vi "RS232 485发送接收.vi"() -> ()   [LabVIEW 2010]
uses:
  全局量/全局_配置.vi
  <vilib>/Instr/_visa.llb/VISA Configure Serial Port (Instr).vi
panel:
  in  "单选_RS485_1":bool
  in  "单选_RS232_2":bool
  in  "单选_RS232_1":bool
  out "接收数据_3":string
  out "成功_3？":bool caption="成功？"
  in  "发送数据_3":string
  out "接收数据_2":string
  out "成功_2？":bool caption="成功？"
  in  "发送数据_2":string
  in  "btn_关闭":bool
  in  "btn_开始测试":bool
  out "接收数据_1":string
  out "成功_1？":bool caption="成功？"
  in  "发送数据_1":string
  # "RS232测试界面"
  # "1#发送字符"
  # "2#发送字符"
  # "1#接收字符"
  # "2#接收字符"
  # "1#测试结果"
  # "2#测试结果"
  # "RS485测试界面"
  # "1#发送字符"
  # "1#接收字符"
  # "1#测试结果"
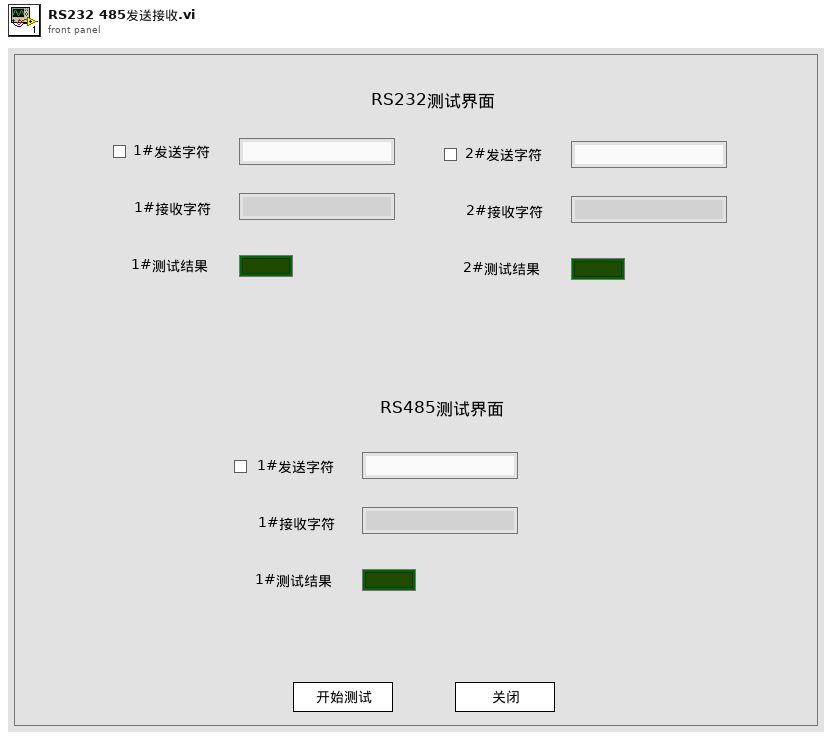
[diagram p1: front panel]
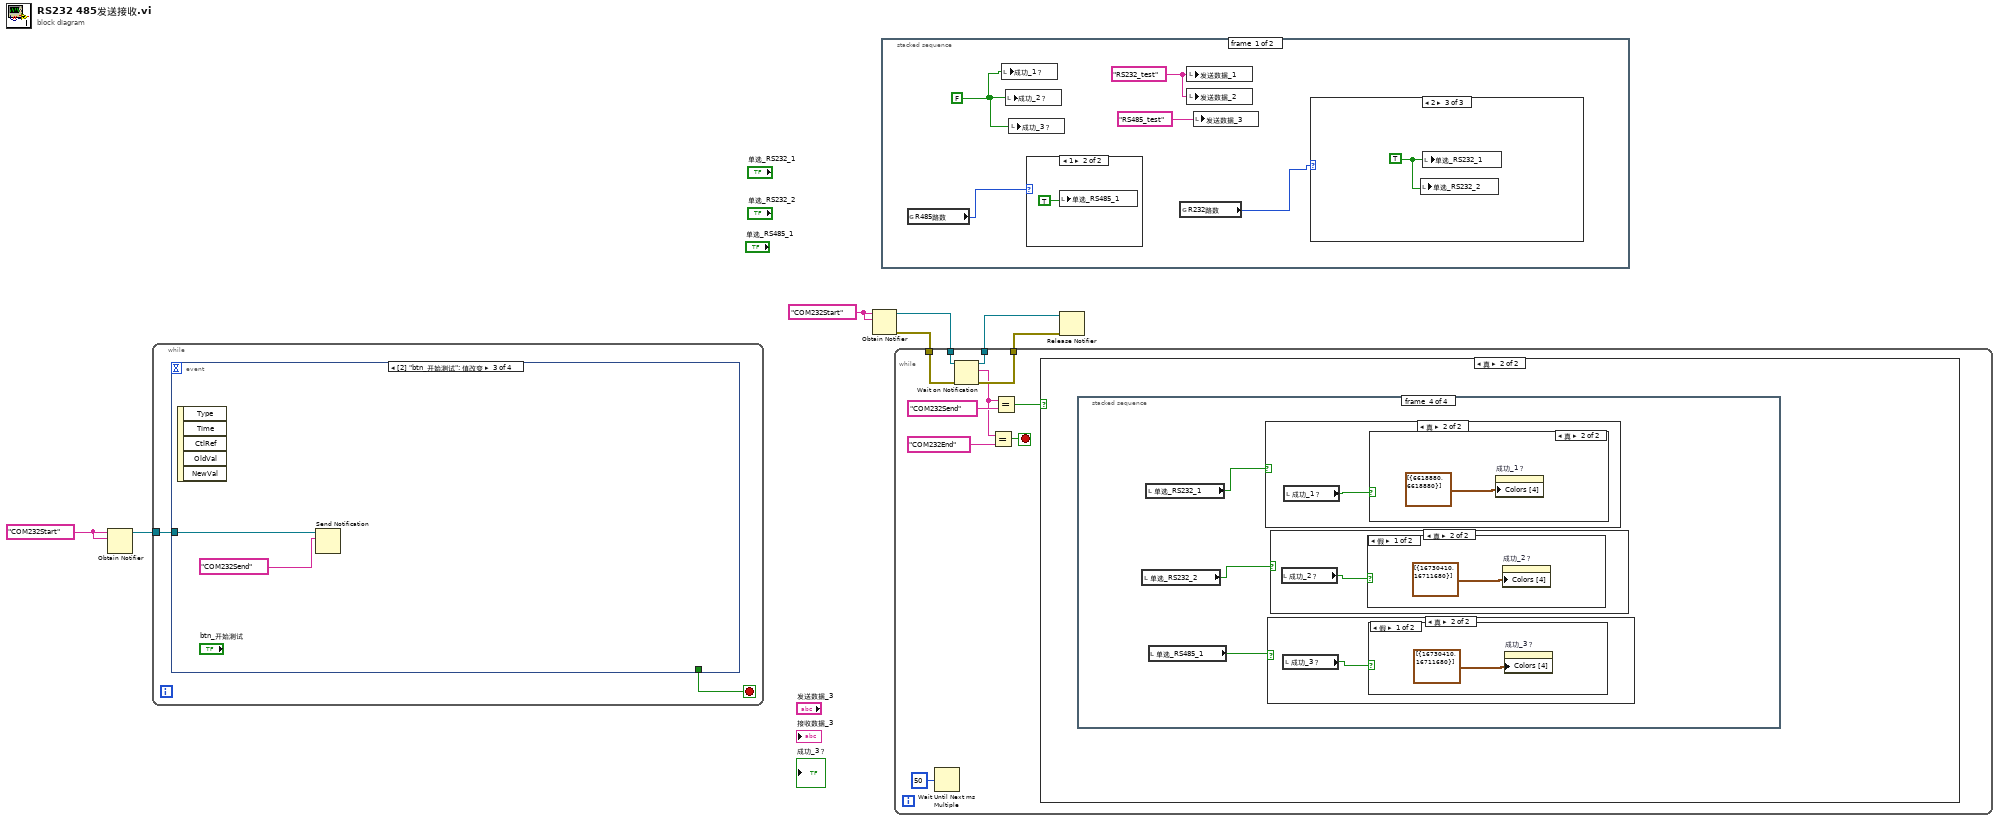
[diagram p0: block diagram]
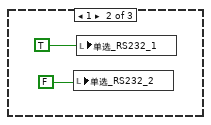
[diagram p3: hidden frame]
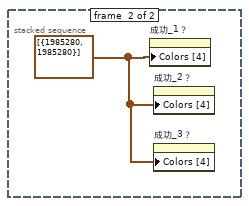
[diagram p5: hidden frame]
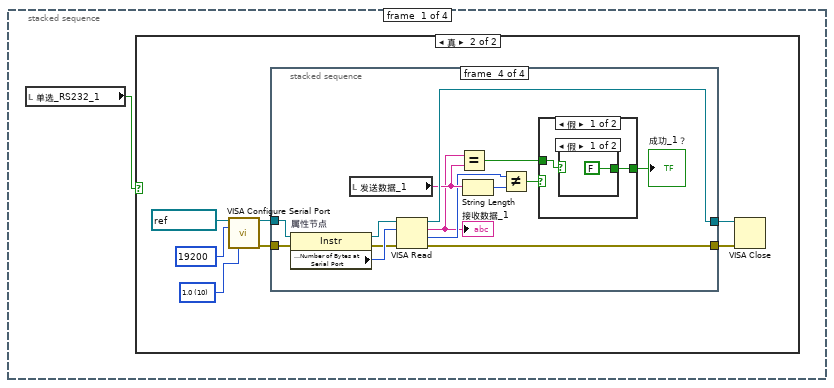
[diagram p7: hidden frame]
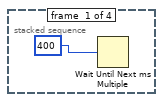
[diagram p9: hidden frame]
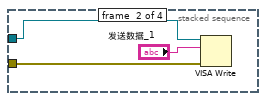
[diagram p10: hidden frame]
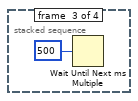
[diagram p11: hidden frame]
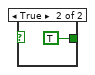
[diagram p12: hidden frame]
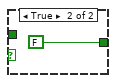
[diagram p13: hidden frame]
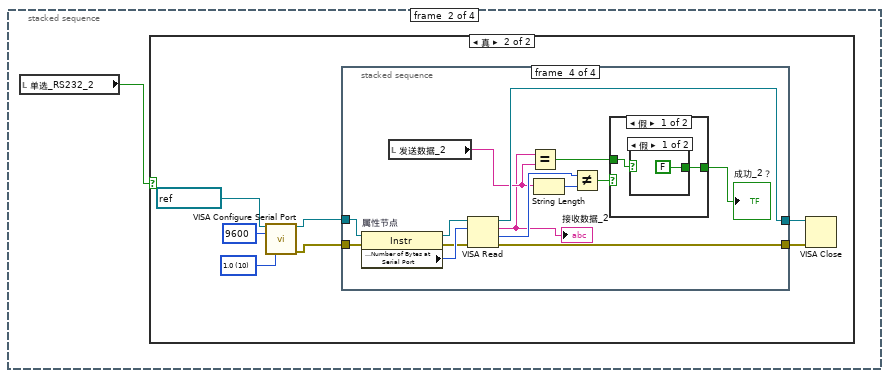
[diagram p14: hidden frame]
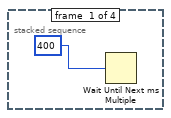
[diagram p16: hidden frame]
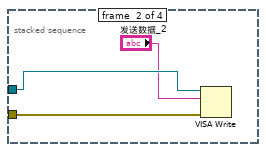
[diagram p17: hidden frame]
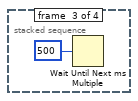
[diagram p18: hidden frame]
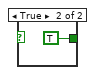
[diagram p19: hidden frame]
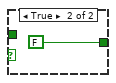
[diagram p20: hidden frame]
diagram:
  w2 = "COM232Start" ("名称（未命名）")
  w7 = "COM232Start" ("名称（未命名）")
  n1 = Obtain Notifier(name (unnamed)=w2, notification data type=w2) -> (notifier out=w1:refnum<notifier>)  [unwired: 2 in, 2 out]
  n2 = while {
    tunnel: w1 -> [w8]
    stop <- w9 stop-if-true
    n3 = event shown="[2] \"btn_开始测试\": 值改变" {
      selector: _ -> [_ _ _ _]
      dyn-events: _ -> [_ _ _ _]
      timeout: _ -> [_ _ _ _]
      tunnel: [_ TRUE _ TRUE] -> w9
      tunnel: w8 -> [_ w11 w13 w15]
      event Timeout {
        n4 = event-data() -> ()  [unwired: 1 in, 2 out]
      }
      event Panel Close {
        n5 = event-data() -> ()  [unwired: 1 in, 3 out]
        n6 = Send Notification(notification="COM232End" ("通知"), notifier=w11) -> ()  [unwired: 1 in, 2 out]
      }
      event "btn_开始测试": Value Change {
        n7 = event-data() -> ()  [unwired: 1 in, 5 out]
        n8 = Send Notification(notification="COM232Send" ("通知"), notifier=w13) -> ()  [unwired: 1 in, 2 out]
      }
      event "btn_关闭": Value Change {
        n9 = event-data() -> ()  [unwired: 1 in, 5 out]
        n10 = Send Notification(notification="COM232End" ("通知"), notifier=w15) -> ()  [unwired: 1 in, 2 out]
      }
    }
  }
  n11 = Obtain Notifier(name (unnamed)=w7, notification data type=w7) -> (notifier out=w6:refnum<notifier>, error out=w5:errorcluster)  [unwired: 2 in, 1 out]
  n12 = stacked-sequence {
    frame #0 {
      w20 = FALSE
      w22 = "RS232_test" ("发送数据_1")
      n13 = global read "全局_配置.vi" "R485路数"() -> (w18:u32)
      n14 = local write "成功_1？"(w20) -> ()
      n15 = local write "成功_2？"(w20) -> ()
      n16 = local write "成功_3？"(w20) -> ()
      n17 = case shown="1" w18 {
        frame 0, Default {
        }
        frame 1 {
          n18 = local write "单选_RS485_1"(TRUE) -> ()
        }
      }
      n19 = global read "全局_配置.vi" "R232路数"() -> (w19:u32)
      n20 = local write "发送数据_1"(w22) -> ()
      n21 = local write "发送数据_2"(w22) -> ()
      n22 = local write "发送数据_3"("RS485_test" ("发送数据_1")) -> ()
      n23 = case shown="2" w19 {
        frame 0, Default {
        }
        frame 1 {
          n24 = local write "单选_RS232_2"(FALSE) -> ()
          n25 = local write "单选_RS232_1"(TRUE) -> ()
        }
        frame 2 {
          w25 = TRUE
          n26 = local write "单选_RS232_2"(w25) -> ()
          n27 = local write "单选_RS232_1"(w25) -> ()
        }
      }
    }
    frame #1 {
      w27 = cluster{u32, u32}[] [{1985280, 1985280}]
      n28 = property on="成功_1？" class="Bool (严格)"("Colors [4]"=w27) -> ()  [unwired: 2 in, 2 out]
      n29 = property on="成功_2？" class="Bool (严格)"("Colors [4]"=w27) -> ()  [unwired: 2 in, 2 out]
      n30 = property on="成功_3？" class="Bool (严格)"("Colors [4]"=w27) -> ()  [unwired: 2 in, 2 out]
    }
  }
  n31 = while {
    tunnel: w6 -> [w37]
    tunnel: w5 -> [w36]
    tunnel: [w35] -> w4
    tunnel: [w34] -> w3
    stop <- w29 stop-if-true
    n32 = Wait Until Next ms Multiple(millisecond multiple=u32 50 ("毫秒倍数")) -> ()  [unwired: 1 out]
    n33 = Wait on Notification(notifier=w37, error in (no error)=w36) -> (notifier out=w35:refnum<notifier>, notification=w31:string, error out=w34:errorcluster)  [unwired: 2 in, 1 out]
    n34 = Equal?(x=w31, y="COM232End" ("通知")) -> (x = y?=w29:bool)
    n35 = Equal?(x=w31, y="COM232Send" ("通知")) -> (x = y?=w32:bool)
    n36 = case shown="真" w32 {
      frame False {
      }
      frame True {
        n37 = stacked-sequence {
          frame #0 {
            n38 = local read "单选_RS232_1"() -> (w38:bool)
            n39 = case shown="真" w38 {
              frame False {
              }
              frame True {
                w43 = u16 10 items=["1.0"=10, "1.5"=15, "2.0"=20] ("stop bits (10: 1 bit)")
                n40 = call-poly "VISA Configure Serial Port"("VISA resource name"=refnum<visa-resource-name> "COM1" ("R232端口"), "baud rate (9600)"=u32 19200, "stop bits (10: 1 bit)"=w43) -> ("VISA resource name out"=w42:refnum<visa-resource-name>, "error out"=w41:errorcluster)  [unwired: 11 in]
                n41 = stacked-sequence {
                  tunnel: w42 -> [_ w49 _ w62]
                  tunnel: w41 -> [_ w48 _ w61]
                  tunnel: [_ _ _ w64] -> w40
                  tunnel: [_ _ _ w63] -> w39
                  frame #0 {
                    n42 = Wait Until Next ms Multiple(millisecond multiple=u32 400 ("毫秒倍数")) -> ()  [unwired: 1 out]
                  }
                  frame #1 {
                    n43 = VISA Write(VISA resource name=w49, write buffer="发送数据_1", error in (no error)=w48) -> ()  [unwired: 3 out]
                  }
                  frame #2 {
                    n44 = Wait Until Next ms Multiple(millisecond multiple=u32 500 ("毫秒倍数")) -> ()  [unwired: 1 out]
                  }
                  frame #3 {
                    n45 = property on="属性节点" class="Instr"(reference=w62, error in=w61) -> (reference out=w58:refnum<visa-resource-name>, error out=w56:errorcluster, "Serial Settings:Number of Bytes at Serial Port"=w57:u32)
                    n46 = local read "发送数据_1"() -> (w55:string)
                    n47 = VISA Read(VISA resource name=w58, byte count=w57, error in (no error)=w56) -> (VISA resource name out=w64:refnum<visa-resource-name>, read buffer=w51:string, return count=w54:u32, error out=w63:errorcluster)
                    "接收数据_1" <- w51
                    n48 = Equal?(x=w51, y=w55) -> (x = y?=w60:bool)
                    n49 = String Length(string=w55) -> (length=w53:i32)
                    n50 = Not Equal?(x=w54, y=w53) -> (x != y?=w52:bool)
                    n51 = case shown="假" w52 {
                      tunnel: w60 -> [w66 _]
                      tunnel: [w65 FALSE] -> w59
                      frame False {
                        n52 = case shown="假" w66 {
                          tunnel: [FALSE TRUE] -> w65
                          frame False {
                          }
                          frame True {
                          }
                        }
                      }
                      frame True {
                      }
                    }
                    "成功_1？" <- w59
                  }
                }
                n53 = VISA Close(VISA resource name=w40, error in (no error)=w39) -> ()  [unwired: 1 out]
              }
            }
          }
          frame #1 {
            n54 = local read "单选_RS232_2"() -> (w70:bool)
            n55 = case shown="真" w70 {
              frame False {
              }
              frame True {
                w75 = u16 10 items=["1.0"=10, "1.5"=15, "2.0"=20] ("stop bits (10: 1 bit)")
                n56 = call-poly "VISA Configure Serial Port"("VISA resource name"=refnum<visa-resource-name> "COM3" ("R232端口"), "baud rate (9600)"=u32 9600, "stop bits (10: 1 bit)"=w75) -> ("VISA resource name out"=w72:refnum<visa-resource-name>, "error out"=w71:errorcluster)  [unwired: 11 in]
                n57 = stacked-sequence {
                  tunnel: w72 -> [_ w81 _ w94]
                  tunnel: w71 -> [_ w80 _ w93]
                  tunnel: [_ _ _ w96] -> w77
                  tunnel: [_ _ _ w95] -> w76
                  frame #0 {
                    n58 = Wait Until Next ms Multiple(millisecond multiple=u32 400 ("毫秒倍数")) -> ()  [unwired: 1 out]
                  }
                  frame #1 {
                    n59 = VISA Write(VISA resource name=w81, write buffer="发送数据_2", error in (no error)=w80) -> ()  [unwired: 3 out]
                  }
                  frame #2 {
                    n60 = Wait Until Next ms Multiple(millisecond multiple=u32 500 ("毫秒倍数")) -> ()  [unwired: 1 out]
                  }
                  frame #3 {
                    n61 = property on="属性节点" class="Instr"(reference=w94, error in=w93) -> (reference out=w91:refnum<visa-resource-name>, error out=w89:errorcluster, "Serial Settings:Number of Bytes at Serial Port"=w90:u32)
                    n62 = local read "发送数据_2"() -> (w85:string)
                    n63 = VISA Read(VISA resource name=w91, byte count=w90, error in (no error)=w89) -> (VISA resource name out=w96:refnum<visa-resource-name>, read buffer=w84:string, return count=w88:u32, error out=w95:errorcluster)
                    "接收数据_2" <- w84
                    n64 = Equal?(x=w84, y=w85) -> (x = y?=w92:bool)
                    n65 = String Length(string=w85) -> (length=w87:i32)
                    n66 = Not Equal?(x=w88, y=w87) -> (x != y?=w86:bool)
                    n67 = case shown="假" w86 {
                      tunnel: w92 -> [w98 _]
                      tunnel: [w97 FALSE] -> w83
                      frame False {
                        n68 = case shown="假" w98 {
                          tunnel: [FALSE TRUE] -> w97
                          frame False {
                          }
                          frame True {
                          }
                        }
                      }
                      frame True {
                      }
                    }
                    "成功_2？" <- w83
                  }
                }
                n69 = VISA Close(VISA resource name=w77, error in (no error)=w76) -> ()  [unwired: 1 out]
              }
            }
          }
          frame #2 {
            n70 = local read "单选_RS485_1"() -> (w102:bool)
            n71 = case shown="真" w102 {
              frame False {
              }
              frame True {
                w107 = u16 10 items=["1.0"=10, "1.5"=15, "2.0"=20] ("stop bits (10: 1 bit)")
                n72 = call-poly "VISA Configure Serial Port"("VISA resource name"=refnum<visa-resource-name> "COM4" ("R232端口"), "baud rate (9600)"=u32 9600, "stop bits (10: 1 bit)"=w107) -> ("VISA resource name out"=w104:refnum<visa-resource-name>, "error out"=w103:errorcluster)  [unwired: 11 in]
                n73 = stacked-sequence {
                  tunnel: w104 -> [_ w113 _ w126]
                  tunnel: w103 -> [_ w112 _ w125]
                  tunnel: [_ _ _ w128] -> w109
                  tunnel: [_ _ _ w127] -> w108
                  frame #0 {
                    n74 = Wait Until Next ms Multiple(millisecond multiple=u32 400 ("毫秒倍数")) -> ()  [unwired: 1 out]
                  }
                  frame #1 {
                    n75 = local read "发送数据_3"() -> (w111:string)
                    n76 = VISA Write(VISA resource name=w113, write buffer=w111, error in (no error)=w112) -> ()  [unwired: 3 out]
                  }
                  frame #2 {
                    n77 = Wait Until Next ms Multiple(millisecond multiple=u32 500 ("毫秒倍数")) -> ()  [unwired: 1 out]
                  }
                  frame #3 {
                    n78 = property on="属性节点" class="Instr"(reference=w126, error in=w125) -> (reference out=w123:refnum<visa-resource-name>, error out=w121:errorcluster, "Serial Settings:Number of Bytes at Serial Port"=w122:u32)
                    n79 = local read "发送数据_3"() -> (w117:string)
                    n80 = VISA Read(VISA resource name=w123, byte count=w122, error in (no error)=w121) -> (VISA resource name out=w128:refnum<visa-resource-name>, read buffer=w116:string, return count=w120:u32, error out=w127:errorcluster)
                    n81 = Equal?(x=w116, y=w117) -> (x = y?=w124:bool)
                    n82 = String Length(string=w117) -> (length=w119:i32)
                    n83 = Not Equal?(x=w120, y=w119) -> (x != y?=w118:bool)
                    n84 = local write "接收数据_3"(w116) -> ()
                    n85 = case shown="假" w118 {
                      tunnel: w124 -> [w130 _]
                      tunnel: [w129 FALSE] -> w115
                      frame False {
                        n86 = case shown="假" w130 {
                          tunnel: [FALSE TRUE] -> w129
                          frame False {
                          }
                          frame True {
                          }
                        }
                      }
                      frame True {
                      }
                    }
                    n87 = local write "成功_3？"(w115) -> ()
                  }
                }
                n88 = VISA Close(VISA resource name=w109, error in (no error)=w108) -> ()  [unwired: 1 out]
              }
            }
          }
          frame #3 {
            n89 = local read "单选_RS232_2"() -> (w135:bool)
            n90 = local read "单选_RS232_1"() -> (w134:bool)
            n91 = local read "单选_RS485_1"() -> (w136:bool)
            n92 = case shown="真" w134 {
              frame False {
              }
              frame True {
                n93 = local read "成功_1？"() -> (w137:bool)
                n94 = case shown="真" w137 {
                  frame False {
                    n95 = property on="成功_1？" class="Bool (严格)"("Colors [4]"=cluster{u32, u32}[] [{16730410, 16711680}]) -> ()  [unwired: 2 in, 2 out]
                  }
                  frame True {
                    n96 = property on="成功_1？" class="Bool (严格)"("Colors [4]"=cluster{u32, u32}[] [{6618880, 6618880}]) -> ()  [unwired: 2 in, 2 out]
                  }
                }
              }
            }
            n97 = case shown="真" w136 {
              frame False {
              }
              frame True {
                n98 = local read "成功_3？"() -> (w143:bool)
                n99 = case shown="假" w143 {
                  frame False {
                    n100 = property on="成功_3？" class="Bool (严格)"("Colors [4]"=cluster{u32, u32}[] [{16730410, 16711680}]) -> ()  [unwired: 2 in, 2 out]
                  }
                  frame True {
                    n101 = property on="成功_3？" class="Bool (严格)"("Colors [4]"=cluster{u32, u32}[] [{6618880, 6618880}]) -> ()  [unwired: 2 in, 2 out]
                  }
                }
              }
            }
            n102 = case shown="真" w135 {
              frame False {
              }
              frame True {
                n103 = local read "成功_2？"() -> (w140:bool)
                n104 = case shown="假" w140 {
                  frame False {
                    n105 = property on="成功_2？" class="Bool (严格)"("Colors [4]"=cluster{u32, u32}[] [{16730410, 16711680}]) -> ()  [unwired: 2 in, 2 out]
                  }
                  frame True {
                    n106 = property on="成功_2？" class="Bool (严格)"("Colors [4]"=cluster{u32, u32}[] [{6618880, 6618880}]) -> ()  [unwired: 2 in, 2 out]
                  }
                }
              }
            }
          }
        }
      }
    }
  }
  n107 = Release Notifier(notifier=w4, error in (no error)=w3) -> ()  [unwired: 1 in, 3 out]
